vi "Stop Processes.vi"(11 "VS Inline Async API in":refnum<class "VS Inline Async API.lvclass">) -> (3 "VS Inline Async API out":refnum<class "VS Inline Async API.lvclass">)   [LabVIEW 2015, in "VS Inline Async API.lvlib" / "VS Inline Async API.lvclass"]
uses:
  VS Inline Async API.lvclass
  VS Inline Async API.lvclass/VS Inline Async API.ctl
  <vilib>/NI Veristand/Custom Device Tools/Custom Device Utility Library/Custom Device Utility Library.lvlib
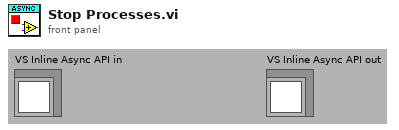
[diagram p1: front panel]
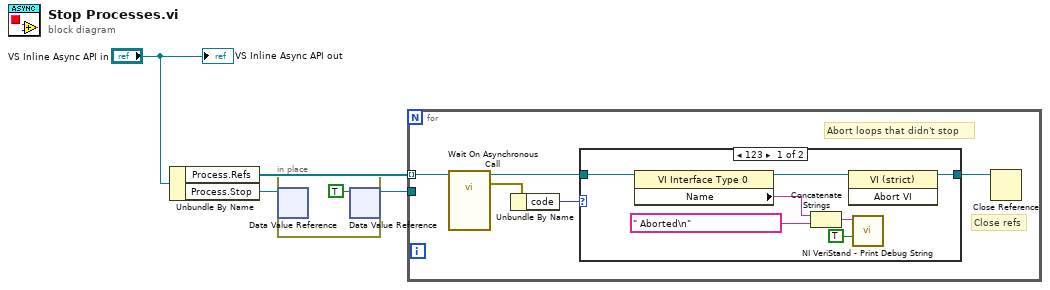
[diagram p0: block diagram]
diagram:
  n1 = Unbundle By Name("VS Inline Async API in") -> ("Process.Refs"=w2:refnum<vi>[], "Process.Stop"=w3:refnum<data-value>)
  n2 = in-place {
    n3 = in-place-dvr #1(w3) -> ()  [unwired: 2 out]
    n4 = in-place-dvr #1(TRUE ("data value")) -> (w1:refnum<data-value>)  [unwired: 1 out]
  }
  n5 = for {
    tunnel: w2 -> [w10] mode=indexing
    tunnel: w1 -> [_]
    # "Close refs"
    # "Abort loops that didn't stop"
    n6 = call-by-ref "Wait On Asynchronous Call"(reference=w10) -> (reference out=w8:refnum<vi>, error out=w7:errorcluster)  [unwired: 13 in]
    n7 = Unbundle By Name(w7) -> ("code"=w6:i32)
    n8 = case shown="123" w6 {
      tunnel: w8 -> [w14 w18]
      tunnel: [w12 w18] -> w9
      frame 123 {
        n9 = property class="VI Interface Type 0"(reference=w14) -> (reference out=w13:refnum<vi>, "Name"=w17:string)  [unwired: 1 in, 1 out]
        n10 = Concatenate Strings(w17, " Aborted\n" ("string")) -> (w15:string)
        n11 = invoke class="VI (strict)" method="Abort VI"(reference=w13) -> (reference out=w12:refnum<vi>)  [unwired: 2 in, 2 out]
        n12 = call <vilib>:"NI VeriStand - Print Debug String.vi"("Add to log file? (T)"=TRUE, "Message"=w15) -> ()  [unwired: 9 in, 1 out]
      }
      frame Default {
      }
    }
    n13 = Close Reference(reference=w9) -> ()  [unwired: 1 in, 1 out]
  }
  "VS Inline Async API out" <- "VS Inline Async API in"
